vi "dataToAscii_8bit.vi"(7 "Pre 3.0 AOM driver version?":bool, 8 "HEX min width (pre 3.0)":u8=2, 9 "Input Data":dbl[](array[numeric]), 10 "Input String":string, 11 "Register":dbl) -> (3 "Characters to FPGA":string)   [LabVIEW 2013, in "DDS9954_v2013.lvlib"]
uses:
  DDS9954_v2013.lvlib
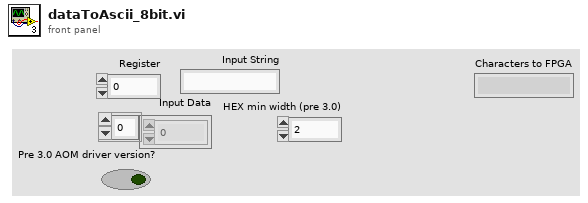
[diagram p1: front panel]
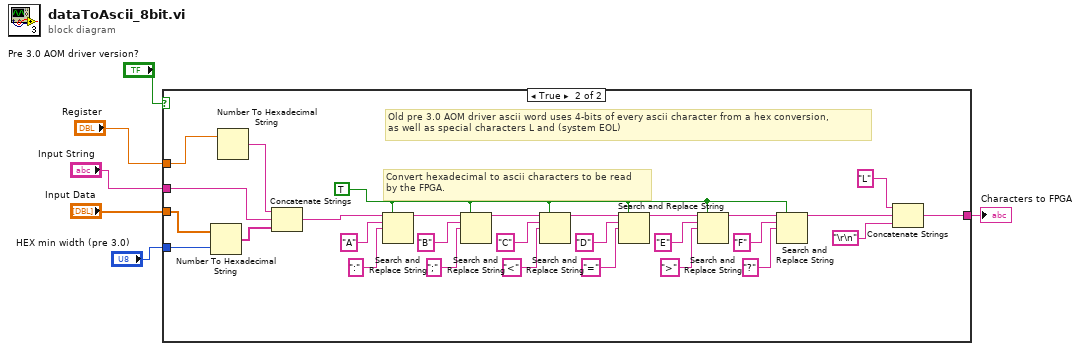
[diagram p0: block diagram]
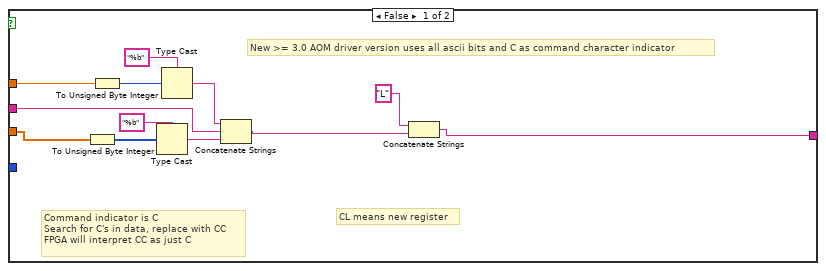
[diagram p2: hidden frame]
diagram:
  n1 = case shown="True" "Pre 3.0 AOM driver version?" {
    tunnel: "Input Data" -> [w13 w47]
    tunnel: "Register" -> [w12 w46]
    tunnel: [w10 w23] -> w4
    tunnel: "Input String" -> [w8 w19]
    tunnel: "HEX min width (pre 3.0)" -> [_ w21]
    frame False {
      # "New >= 3.0 AOM driver version uses all ascii bits and C as command character indicator"
      # "CL means new register"
      # "Command indicator is C\nSearch for C's in data, replace with CC\nFPGA will interpret CC as just C"
      n2 = To Unsigned Byte Integer(number=w13) -> (unsigned 8bit integer=w15:u8[])
      n3 = To Unsigned Byte Integer(number=w12) -> (unsigned 8bit integer=w18:u8)
      n4 = Type Cast(type="%b", x=w15) -> (*(type *) &x=w16:string)
      n5 = Type Cast(type="%b", x=w18) -> (*(type *) &x=w9:string)
      n6 = Concatenate Strings(w9, w8, w16) -> (w7:string)
      n7 = Concatenate Strings("L" ("string"), w7) -> (w10:string)
    }
    frame True {
      w28 = TRUE
      # "Old pre 3.0 AOM driver ascii word uses 4-bits of every ascii character from a hex conversion,\nas well as special characters L and (system EOL)"
      # "Convert hexadecimal to ascii characters to be read\nby the FPGA."
      n8 = Number To Hexadecimal String(1:w21, 2:w47) -> (0:w20:string[])
      n9 = Number To Hexadecimal String(2:w46) -> (0:w26:string)  [unwired: 1 in]
      n10 = Concatenate Strings(w26, w19, w20) -> (w27:string)
      n11 = Search and Replace String(replace all?=w28, input string=w27, search string="A", replace string=":" ("replace string (\"\")")) -> (result string=w33:string)  [unwired: 4 in, 3 out]
      n12 = Search and Replace String(replace all?=w28, input string=w33, search string="B", replace string=";" ("replace string (\"\")")) -> (result string=w32:string)  [unwired: 4 in, 3 out]
      n13 = Search and Replace String(replace all?=w28, input string=w32, search string="C", replace string="<" ("replace string (\"\")")) -> (result string=w31:string)  [unwired: 4 in, 3 out]
      n14 = Search and Replace String(replace all?=w28, input string=w31, search string="D", replace string="=" ("replace string (\"\")")) -> (result string=w30:string)  [unwired: 4 in, 3 out]
      n15 = Search and Replace String(replace all?=w28, input string=w30, search string="E", replace string=">" ("replace string (\"\")")) -> (result string=w29:string)  [unwired: 4 in, 3 out]
      n16 = Search and Replace String(replace all?=w28, input string=w29, search string="F", replace string="?" ("replace string (\"\")")) -> (result string=w24:string)  [unwired: 4 in, 3 out]
      n17 = Concatenate Strings("L" ("string"), w24, "\r\n") -> (w23:string)
    }
  }
  "Characters to FPGA" <- w4
